vi "pix.sgl.CalcPercentiles.vi"(9 "cutoff (%)":T1={"min"=0.0, "max"=100.0}, 10 "number of bins (65536)":i32=65536, 11 "pix":sgl[][](array[numeric])) -> (1 "range":T1, 2 "extrema":T1)   [LabVIEW 2020]
uses:
  _controls/cluster.range.sgl.ctl
  <vilib>/Analysis/NI_AALBase.lvlib
panel:
  out "# in lower":u32
  out "# in upper":u32
  # "This VI replaces the old \"pix.sgl.CalcPercentiles.sgl.core\". \nOur roll-your-own histogram is no where near as fast as \nthe LV native version (maybe LV got a recent boost?), \nso we now use the speedy version here!"
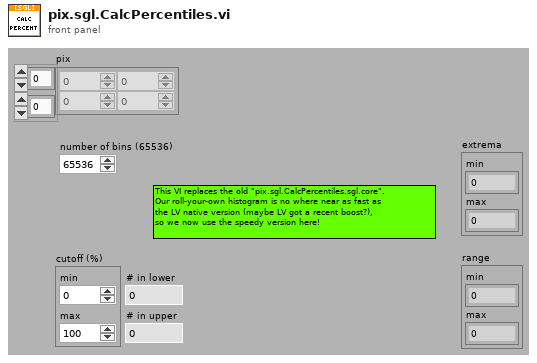
[diagram p1: front panel]
types:
  T1 = typedef "cluster.range.sgl.ctl" = cluster{"min":sgl, "max":sgl}
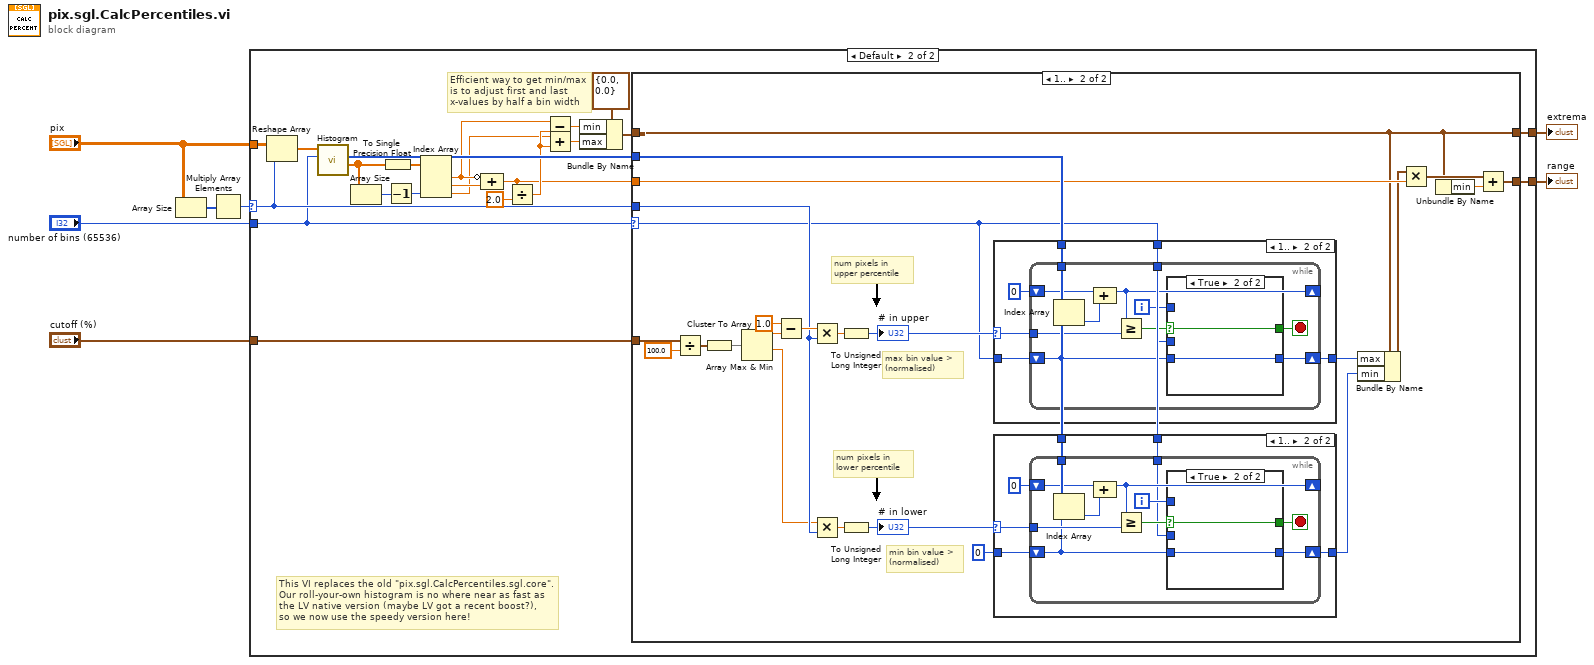
[diagram p0: block diagram]
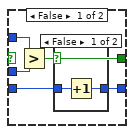
[diagram p5: hidden frame]
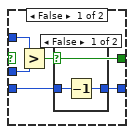
[diagram p8: hidden frame]
diagram:
  n1 = Array Size(array="pix") -> (size(s)=w5:i32[])
  n2 = Multiply Array Elements(1:w5) -> (0:w4:i32)
  n3 = case shown="Default" w4 {
    selector: w4 -> [_ w26]
    tunnel: "pix" -> [_ w25]
    tunnel: "cutoff (%)" -> [_ w27]
    tunnel: "number of bins (65536)" -> [_ w16]
    tunnel: [_ w28] -> w3
    tunnel: [_ w29] -> w2
    frame 0 {
      # "Invalid input image:\n - Return zero range"
    }
    frame Default {
      # "This VI replaces the old \"pix.sgl.CalcPercentiles.sgl.core\". \nOur roll-your-own histogram is no where near as fast as \nthe LV native version (maybe LV got a recent boost?), \nso we now use the speedy version here!"
      # "Efficient way to get min/max \nis to adjust first and last \nx-values by half a bin width"
      n4 = Reshape Array(w25, w26) -> (w18:sgl[])
      n5 = call <vilib>:"Histogram.vi"("intervals"=w16, "X"=w18) -> ("X Values"=w20:dbl[], "Histogram: h(x)"=w24:i32[])  [unwired: 6 in, 2 out]
      n6 = Array Size(array=w20) -> (size(s)=w23:i32)
      n7 = To Single Precision Float(number=w20) -> (single precision float=w9:sgl[])
      n8 = Decrement(x=w23) -> (x-1=w12:i32)
      n9 = Index Array(array=w9, index #3=w12) -> (element #1=w13:sgl, element #2=w17:sgl, element #3=w10:sgl)  [unwired: 2 in]
      n10 = Compound Arithmetic op=ADD(invert w13, w17) -> (w11:sgl)
      n11 = Divide(x=w11, y=sgl 2.0) -> (x/y=w19:sgl)
      n12 = Subtract(x=w13, y=w19) -> (x-y=w14:sgl)
      n13 = Add(x=w10, y=w19) -> (x+y=w15:sgl)
      n14 = Bundle By Name(cluster=T1 {"min"=0.0, "max"=0.0} ("extrema"), "min"=w14, "max"=w15) -> (w22:T1)
      n15 = case shown="1.." w16 {
        selector: w16 -> [_ w37]
        tunnel: w26 -> [_ w42]
        tunnel: w22 -> [w30 w32]
        tunnel: [w30 w51] -> w29
        tunnel: [w30 w32] -> w28
        tunnel: w27 -> [_ w40]
        tunnel: w24 -> [_ w39]
        tunnel: w11 -> [_ w38]
        frame Default {
          # "Illegal number of bins:\n - Return full range"
        }
        frame 1.. {
          # "max bin value >\n(normalised)"
          # "min bin value >\n(normalised)"
          # "num pixels in \nlower percentile"
          # "num pixels in \nupper percentile"
          n16 = Divide(x=w40, y=sgl 100.0 ("max")) -> (x/y=w34:T1)
          n17 = Cluster To Array(cluster=w34) -> (array=w33:sgl[])
          n18 = Array Max & Min(array=w33) -> (max value=w36:sgl, min value=w35:sgl)  [unwired: 2 out]
          n19 = Subtract(x=sgl 1.0, y=w36) -> (x-y=w48:sgl)
          n20 = Multiply(x=w48, y=w42) -> (x*y=w49:sgl)
          n21 = Multiply(x=w35, y=w42) -> (x*y=w47:sgl)
          n22 = To Unsigned Long Integer(number=w49) -> (unsigned 32bit integer=w46:u32)
          "# in upper" <- w46
          n23 = To Unsigned Long Integer(number=w47) -> (unsigned 32bit integer=w44:u32)
          "# in lower" <- w44
          n24 = case shown="1.." w46 {
            selector: w46 -> [_ w85]
            tunnel: w39 -> [_ w89]
            tunnel: [w83 w86] -> w54
            tunnel: w37 -> [w83 w87]
            tunnel: w37 -> [_ w84]
            frame ..0 {
            }
            frame 1.. {
              n25 = while {
                tunnel: w89 -> [w100]
                tunnel: w85 -> [w99]
                shift-right: [w98] -> w86
                shift-left: w87 -> [w96]
                shift-right: [w94] -> _
                shift-left: u32 0 ("element") -> [w97]
                tunnel: w84 -> [w90]
                i -> [w92]
                stop <- w91 stop-if-true
                n26 = Index Array(array=w100, index=w96) -> (element=w95:i32)
                n27 = Compound Arithmetic op=ADD(w97, w95) -> (w94:u32)
                n28 = Greater Or Equal?(x=w94, y=w99) -> (x >= y?=w93:bool)
                n29 = case shown="True" w93 {
                  selector: w93 -> [_ w110]
                  tunnel: [w105 w109] -> w98
                  tunnel: w96 -> [w104 w109]
                  tunnel: w92 -> [w103 _]
                  tunnel: w90 -> [w102 _]
                  tunnel: [w101 w110] -> w91
                  frame False {
                    n30 = Greater?(x=w103, y=w102) -> (0:w101:bool)
                    n31 = case shown="False" w101 {
                      tunnel: [w107 w108] -> w105
                      tunnel: w104 -> [w106 w108]
                      frame False {
                        n32 = Decrement(x=w106) -> (x-1=w107:i32)
                      }
                      frame True {
                      }
                    }
                  }
                  frame True {
                  }
                }
              }
            }
          }
          n33 = case shown="1.." w44 {
            selector: w44 -> [_ w58]
            tunnel: w39 -> [_ w60]
            tunnel: [w55 w59] -> w53
            tunnel: 0 ("min") -> [w55 w57]
            tunnel: w37 -> [_ w56]
            frame ..0 {
            }
            frame 1.. {
              n34 = while {
                tunnel: w60 -> [w72]
                tunnel: w58 -> [w71]
                shift-right: [w70] -> w59
                shift-left: w57 -> [w68]
                shift-right: [w66] -> _
                shift-left: u32 0 ("element") -> [w69]
                tunnel: w56 -> [w62]
                i -> [w64]
                stop <- w63 stop-if-true
                n35 = Index Array(array=w72, index=w68) -> (element=w67:i32)
                n36 = Compound Arithmetic op=ADD(w69, w67) -> (w66:u32)
                n37 = Greater Or Equal?(x=w66, y=w71) -> (x >= y?=w65:bool)
                n38 = case shown="True" w65 {
                  selector: w65 -> [_ w81]
                  tunnel: [w77 w82] -> w70
                  tunnel: w68 -> [w76 w82]
                  tunnel: w64 -> [w75 _]
                  tunnel: w62 -> [w74 _]
                  tunnel: [w73 w81] -> w63
                  frame False {
                    n39 = Greater?(x=w75, y=w74) -> (0:w73:bool)
                    n40 = case shown="False" w73 {
                      tunnel: [w79 w80] -> w77
                      tunnel: w76 -> [w78 w80]
                      frame False {
                        n41 = Increment(x=w78) -> (x+1=w79:i32)
                      }
                      frame True {
                      }
                    }
                  }
                  frame True {
                  }
                }
              }
            }
          }
          n42 = Bundle By Name(cluster=w32, "max"=w54, "min"=w53) -> (w31:T1)
          n43 = Multiply(x=w31, y=w38) -> (x*y=w52:T1)
          n44 = Unbundle By Name(w32) -> ("min"=w43:sgl)
          n45 = Add(x=w52, y=w43) -> (x+y=w51:T1)
        }
      }
    }
  }
  "extrema" <- w3
  "range" <- w2
